vi "TweakMotorPosition.vi"(11 "Topas":refnum<k24>) -> (3 "Topas Out":refnum<k24>)   [LabVIEW 2014]
doc: "Shows how move single motor to desired position and get information about motor."
uses:
  D:/c#/c#projects/Topas4PublicAPI/NET_SDK/Topas4Lib.dll
  NET_SDK/Topas4Lib.dll
panel:
  in  "Step size":i32=8
  out "Title":string
  out "ActualPosition":i32
  out "TargetPosition":i32
  in  "stop":bool
  in  "Finish":bool
  in  "Forward":bool
  in  "Back":bool
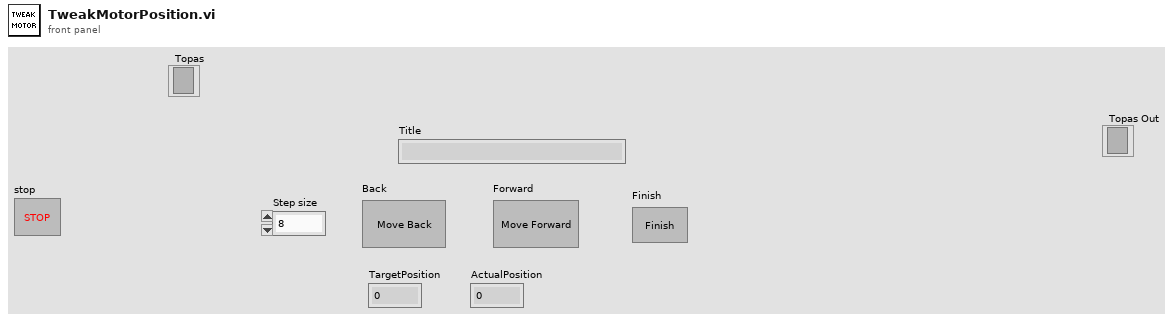
[diagram p1: front panel]
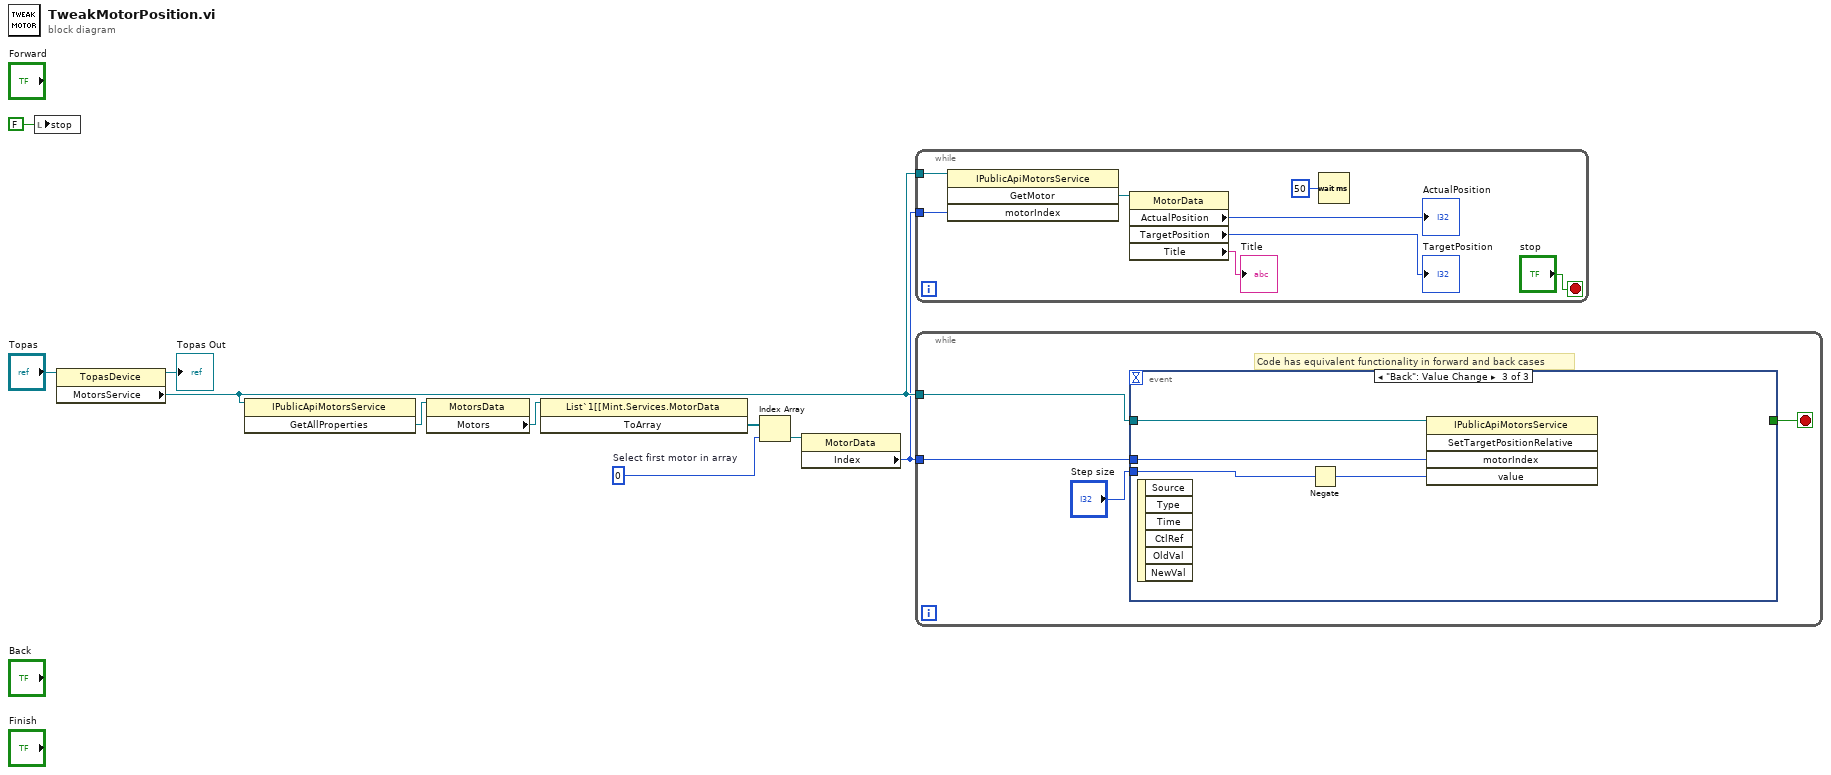
[diagram p0: block diagram]
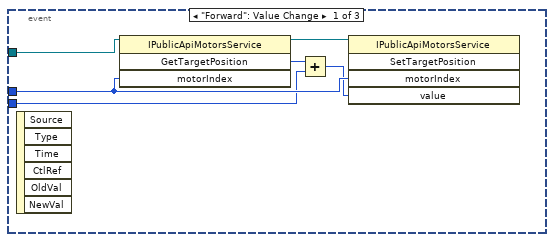
[diagram p2: hidden frame]
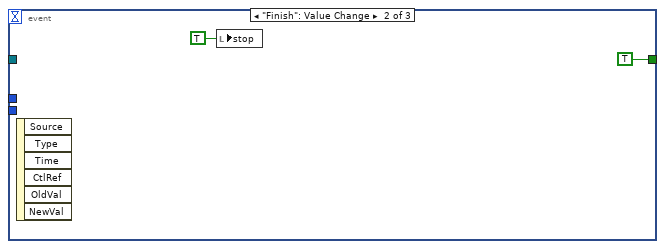
[diagram p3: hidden frame]
diagram:
  w6 = 0  # Select first motor in array
  n1 = local write "stop"(FALSE ("stop")) -> ()
  n2 = property class="TopasDevice"(reference="Topas") -> (reference out=→"Topas Out":refnum<k24>, "MotorsService"=w2:refnum<k24>)  [unwired: 1 in, 1 out]
  n3 = invoke class="IPublicApiMotorsService" method="GetAllProperties"(reference=w2) -> ("GetAllProperties"=w9:refnum<k24>)  [unwired: 2 in, 2 out]
  n4 = property class="MotorsData"(reference=w9) -> ("Motors"=w8:refnum<k24>)  [unwired: 1 in, 2 out]
  n5 = invoke class="List`1[[Mint.Services.MotorData" method="ToArray"(reference=w8) -> ("ToArray"=w7:refnum<k24>[])  [unwired: 2 in, 2 out]
  n6 = Index Array(array=w7, index=w6) -> (element=w5:refnum<k24>)
  n7 = property class="MotorData"(reference=w5) -> ("Index"=w1:i32)  [unwired: 1 in, 2 out]
  n8 = while {
    tunnel: w2 -> [w17]
    tunnel: w1 -> [w16]
    stop <- "stop" stop-if-true
    n9 = invoke class="IPublicApiMotorsService" method="GetMotor"(reference=w17, "motorIndex"=w16) -> ("GetMotor"=w15:refnum<k24>)  [unwired: 2 in, 3 out]
    n10 = property class="MotorData"(reference=w15) -> ("ActualPosition"=→"ActualPosition":i32, "TargetPosition"=→"TargetPosition":i32, "Title"=→"Title":string)  [unwired: 1 in, 2 out]
    n11 = Wait (ms)(milliseconds to wait=u32 50) -> ()  [unwired: 1 out]
  }
  n12 = while {
    tunnel: w1 -> [w21]
    tunnel: w2 -> [w20]
    stop <- w19 stop-if-true
    # "Code has equivalent functionality in forward and back cases"
    n13 = event shown="[2] \"Back\": Value Change" {
      selector: _ -> [_ _ _]
      dyn-events: _ -> [_ _ _]
      timeout: _ -> [_ _ _]
      tunnel: w21 -> [w28 _ w34]
      tunnel: "Step size" -> [w25 _ w33]
      tunnel: w20 -> [w23 _ w31]
      tunnel: [_ TRUE _] -> w19
      event "Forward": Value Change {
        n14 = event-data() -> ()  [unwired: 1 in, 6 out]
        n15 = invoke class="IPublicApiMotorsService" method="GetTargetPosition"(reference=w23, "motorIndex"=w28) -> (reference out=w24:refnum<k24>, "GetTargetPosition"=w27:i32)  [unwired: 2 in, 2 out]
        n16 = Add(x=w27, y=w25) -> (x+y=w26:i32)
        n17 = invoke class="IPublicApiMotorsService" method="SetTargetPosition"(reference=w24, "motorIndex"=w28, "value"=w26) -> ()  [unwired: 2 in, 5 out]
      }
      event "Finish": Value Change {
        n18 = event-data() -> ()  [unwired: 1 in, 6 out]
        n19 = local write "stop"(TRUE ("stop")) -> ()
      }
      event "Back": Value Change {
        n20 = event-data() -> ()  [unwired: 1 in, 6 out]
        n21 = Negate(x=w33) -> (-x=w32:i32)
        n22 = invoke class="IPublicApiMotorsService" method="SetTargetPositionRelative"(reference=w31, "motorIndex"=w34, "value"=w32) -> ()  [unwired: 2 in, 5 out]
      }
    }
  }
